vi "USERCallVISample-IMAQDisplay.vi"(4 "Thread No.":u32, 5 "ProgramRef":refnum<vi>, 6 "Thread Mod Recive":refnum<queue>[](array[refnum]), 7 "ThreadsQueue":refnum<queue>[](array[refnum]), 8 "ThreadInfoIN":T2, 10 "StackIn":cluster{"Program":i32, "Prog Index":i32}[](array[cluster]), 11 "PrameterS":string) -> (0 "ThreadInfoOut":T2, 2 "StackOut":cluster{"Program":i32, "Prog Index":i32}[](array[cluster]), 3 "ErrorCode":string)   [LabVIEW 2020]
panel:
  out "Image":T1(plugin-control)
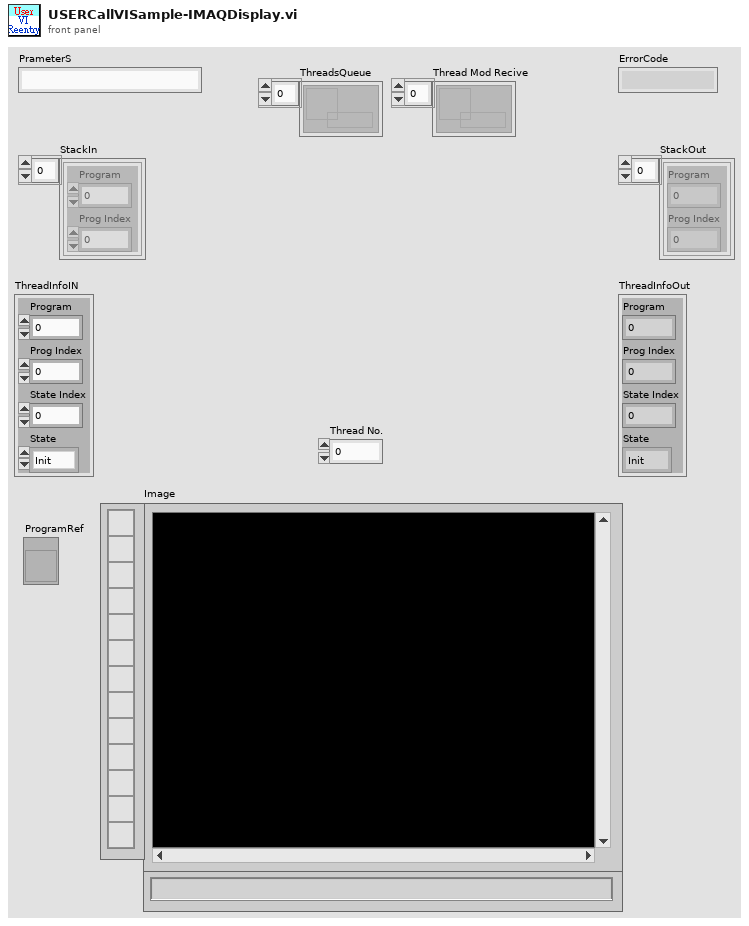
[diagram p1: front panel]
types:
  T1 = typedef "IMAQ Image.ctl" = refnum<image>
  T2 = cluster{"Program":i32, "Prog Index":i32, "State Index":i32, "State":enum16{"Init", "Idle", "Auto Start", "Auto Running", "Step Start", "Step Running", "Suspend", "Restart", "Stop", "Reset"}}
  T3 = cluster{"Global Rectangle":i32[], "Contours":cluster{"Contour Type":u32, "ROI Type":u32, "Points":i32[]}[]}
  T4 = enum16{"Init", "Idle", "Auto Start", "Auto Running", "Step Start", "Step Running", "Suspend", "Restart", "Stop", "Reset"}
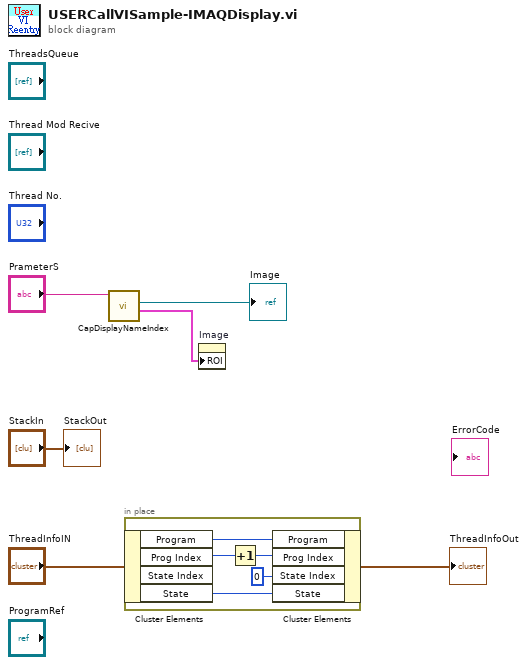
[diagram p0: block diagram]
diagram:
  n1 = call "CapDisplayNameIndex.vi"("CamName"="PrameterS") -> ("ROI"=w3:T3, "IMAQ"=→"Image":T1)  [unwired: 4 in, 2 out]
  n2 = in-place {
    n3 = in-place-cluster #1("ThreadInfoIN") -> ("Program"=w11:i32, "Prog Index"=w9:i32, "State"=w7:T4)  [unwired: 1 out]
    n4 = Increment(x=w9) -> (x+1=w10:i32)
    n5 = in-place-cluster #1("Program"=w11, "Prog Index"=w10, "State Index"=0, "State"=w7) -> (→"ThreadInfoOut":T2)
  }
  n6 = property on="Image" class="ImageControl"("ROI"=w3) -> ()  [unwired: 2 in, 2 out]
  "StackOut" <- "StackIn"
